vi "FTW-Test-CSV-2DArray.vi"() -> ()   [LabVIEW 2015]
panel:
  out "CSV String":string
  out "error out":errorcluster
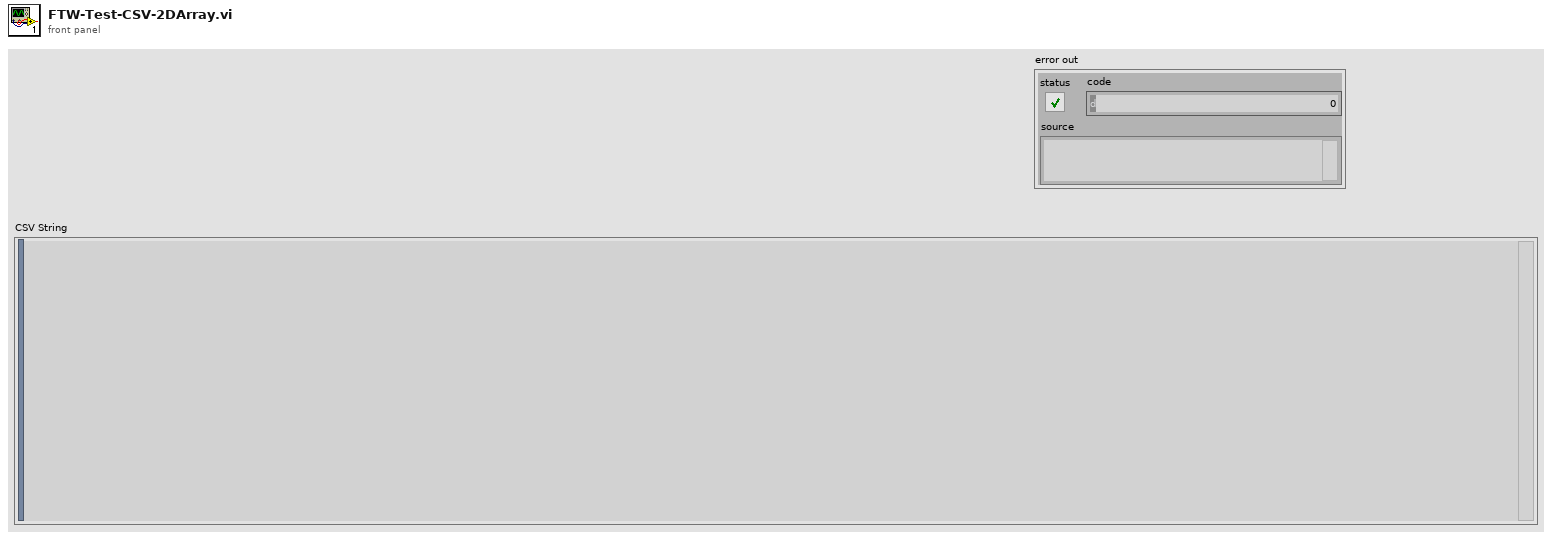
[diagram p1: front panel]
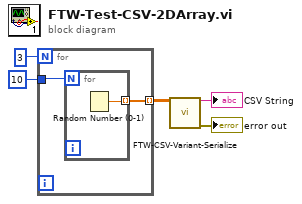
[diagram p0: block diagram]
diagram:
  n1 = for {
    N: 3 -> [_]
    tunnel: 10 -> [w7]
    tunnel: [w6] -> w2 mode=indexing
    n2 = for {
      N: w7 -> [_]
      tunnel: [w8] -> w6 mode=indexing
      n3 = Random Number (0-1)() -> (number: 0 to 1=w8:dbl)
    }
  }
  n4 = call "FTW-CSV-Variant-Serialize.vi"("Variant"=w2) -> ("CSV String"=→"CSV String":string, "error out"=→"error out":errorcluster)  [unwired: 13 in]
